vi "getAUX.vi"(8 "error in (no error)":errorcluster, 10 "Channel":i32=1 min=1 max=16, 11 "Instrument.LockinAPI in":refnum<class "Instrument.LockinAPI.lvclass">) -> (0 "error out":errorcluster, 2 "AUX (V)":dbl, 3 "Instrument.LockinAPI out":refnum<class "Instrument.LockinAPI.lvclass">)   [LabVIEW 2019, in "Instrument.LockinAPI.lvclass"]
doc: "API to get the AO waveforms.\n\nIf address=\"\", this API reads from localhost\nIf address is remote lockin, you need to add this computer to allowed whitelist on the lockin computer you are trying to access."
uses:
  Instrument.LockinAPI.lvclass
  C:/Users/patrick/Documents/GitHub/Instrument-Framework/lvsrc/Instrument/Instrument.lvclass
  Typedefs/API/LockinAPI.Commands--Enum.ctl
  b38456d9-8de6-4f7a-99f9-40c3abb8b43e.vi
  b38456d9-8de6-4f7a-99f9-40c3abb8b43e.vi/aa4066c2-9c52-49bb-a2a5-25bb29cc04b3.vi
  b38456d9-8de6-4f7a-99f9-40c3abb8b43e.vi/aa4066c2-9c52-49bb-a2a5-25bb29cc04b3.vi/18005be5-aa1f-4c56-8451-28c64ec36a18.vi
  b38456d9-8de6-4f7a-99f9-40c3abb8b43e.vi/aa4066c2-9c52-49bb-a2a5-25bb29cc04b3.vi/fd35e9d2-490b-48ad-8c5a-b405da520fba.vi
  b38456d9-8de6-4f7a-99f9-40c3abb8b43e.vi/aa4066c2-9c52-49bb-a2a5-25bb29cc04b3.vi/b6620a27-a3c8-42a1-8d7e-540682ce922b.vi
  <vilib>/JDP Science/JSONtext/Make JSON Array.vi
  b38456d9-8de6-4f7a-99f9-40c3abb8b43e.vi/aa4066c2-9c52-49bb-a2a5-25bb29cc04b3.vi/fd35e9d2-490b-48ad-8c5a-b405da520fba.vi/c2f7ee20-4b8e-4f71-9077-300957d23885.vi
  b38456d9-8de6-4f7a-99f9-40c3abb8b43e.vi/aa4066c2-9c52-49bb-a2a5-25bb29cc04b3.vi/b6620a27-a3c8-42a1-8d7e-540682ce922b.vi/200b80d7-1278-4619-b127-f4d15b14ddea.vi
  b38456d9-8de6-4f7a-99f9-40c3abb8b43e.vi/aa4066c2-9c52-49bb-a2a5-25bb29cc04b3.vi/b6620a27-a3c8-42a1-8d7e-540682ce922b.vi/0b0c40dc-c4c7-499e-8149-219bf4c60dad.vi
  Instrument/API/Enum to String.vi
  Instrument/Private/Get RC Connection Status.vi
  <vilib>/JDP Science/JSONtext/Variant to JSON Text.vi
  <vilib>/JDP Science/JSONtext/support/Format JSON Array Text.vi
  Instrument/API/Send and Receive.vi
  <vilib>/JDP Science/JSONtext/JSON text to Variant.vi
  <vilib>/Utility/Data Type/Get Type Information.vi
  <vilib>/JDP Science/JSONtext/LVClass Serializer/JSONtext LVClass Serializer.lvclass
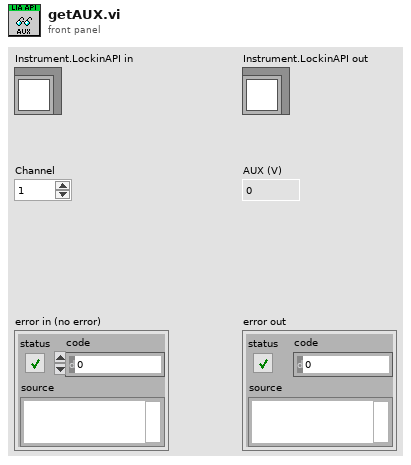
[diagram p1: front panel]
types:
  T1 = typedef "Instrument.LockinAPI.lvclass/LockinAPI.Commands--Enum.ctl" = enum16{"setAI", "setAO", "setAO_Amplitude", "setAO_DC", "setAO_Frequency", "setAO_Phase", "setAO_Function", "setAO_I+", "setREF", "setREF_Frequency", "setREF_Phase", "setREF_TC", "setREF_Roll-Off", "setDAQ", "setSampling", "setOffset", "setState", "getState", "getAO", "getAI", "getResults", "getSampling", "getAOconfig", "getREFconfig", "setInputGain", "setOutputGain", "getInputGain", "getOutputGain", "setSamplingMode", "getSamplingMode", "setSweep", "setSweepTime", "setSweepTable", "getStatus", "getSweepResults", "getSweepWaveforms", "startSweep", "stopSweep", "setAUX", "getAUX"}
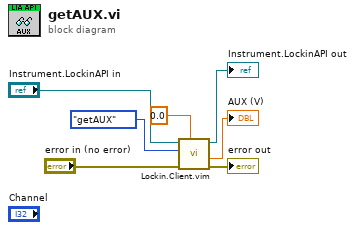
[diagram p0: block diagram]
diagram:
  n1 = call "Lockin.Client.vim"("Data Out type"=0.0 ("AUX (V)"), "error in (no error)"="error in (no error)", "Command"=LockinAPI.Commands--Enum."getAUX", "Instrument.LockinAPI in"="Instrument.LockinAPI in") -> ("error out"=→"error out":errorcluster, "Data out"=→"AUX (V)":dbl, "Instrument.LockinAPI out"=→"Instrument.LockinAPI out":refnum<class "Instrument.LockinAPI.lvclass">)  [unwired: 5 in]
